vi "Calabro_10566859.vi"() -> ()   [LabVIEW 2017]
uses:
  <vilib>/sound2/lvsound2.llb/Sound Data Format.ctl
  <vilib>/sound2/lvsound2.llb/Sampling Mode.ctl
  <extravilib>/ChannelInstances/Stream-a[.](wfm(dbl))/Read With Abort.vi
  <extravilib>/ChannelInstances/Stream-a[.](wfm(dbl))/Write With Abort.vi
  <extravilib>/ChannelInstances/Stream-a[.](wfm(dbl))/EndpointRead.vi
  <extravilib>/ChannelInstances/Stream-a[.](wfm(dbl))/Endpoint.vi
  <vilib>/sound2/lvsound2.llb/Sound Output Write (DBL Single).vi
  <vilib>/sound2/lvsound2.llb/Sound File Write Open.vi
  <extravilib>/ChannelInstances/Stream-a[.](wfm(dbl))/Instantiate.vi
  <extravilib>/ChannelInstances/Stream-a[.](wfm(dbl))/)Channel.vi
  <resource>/ChannelSupport/_ChannelSupport/WaitIfNeeded.vi
  <vilib>/sound2/lvsound2.llb/Sound File Write (DBL).vi
  <vilib>/measure/matone.llb/Extract Single Tone Information N Chan.vi
  <vilib>/sound2/lvsound2.llb/Sound Input Read (DBL).vi
  <vilib>/measure/NI_MABase.lvlib
  <extravilib>/ChannelInstances/Stream-a[.](wfm(dbl)).lvlib
  <vilib>/measure/NI_MAPro.lvlib
panel:
  in  ".WAV file path":path
  in  "Save audio":bool
  out "Acquired sig. frequency":dbl[](array[numeric]) format="%.2p"
  out "Generated sinusoid":waveform(dbl)(graph)
  in  "Sinusoid generation":bool
  in  "Amplitude (V)":dbl(slide) scale=0.0..10.0
  in  "Frequency (Hz)":dbl(knob) scale=0.0..10000.0
  out "Acquired Audio Graph":waveform(dbl)[](graph)
  in  "stop":bool
  # "Name: Davide Calabrò\nPerson Code: 10566859\nMatricola: 944490"
  # "Exercise 1"
  # "I assume the amplitude expressed in\nvolts (V). I don't know how my sound\ncard manages it."
  # "Exercise 2"
  # "In this exercise I also add a waveform graph\njust to visualize the created sinusoid"
  # "Exercise 3"
  # "Exercise 4"
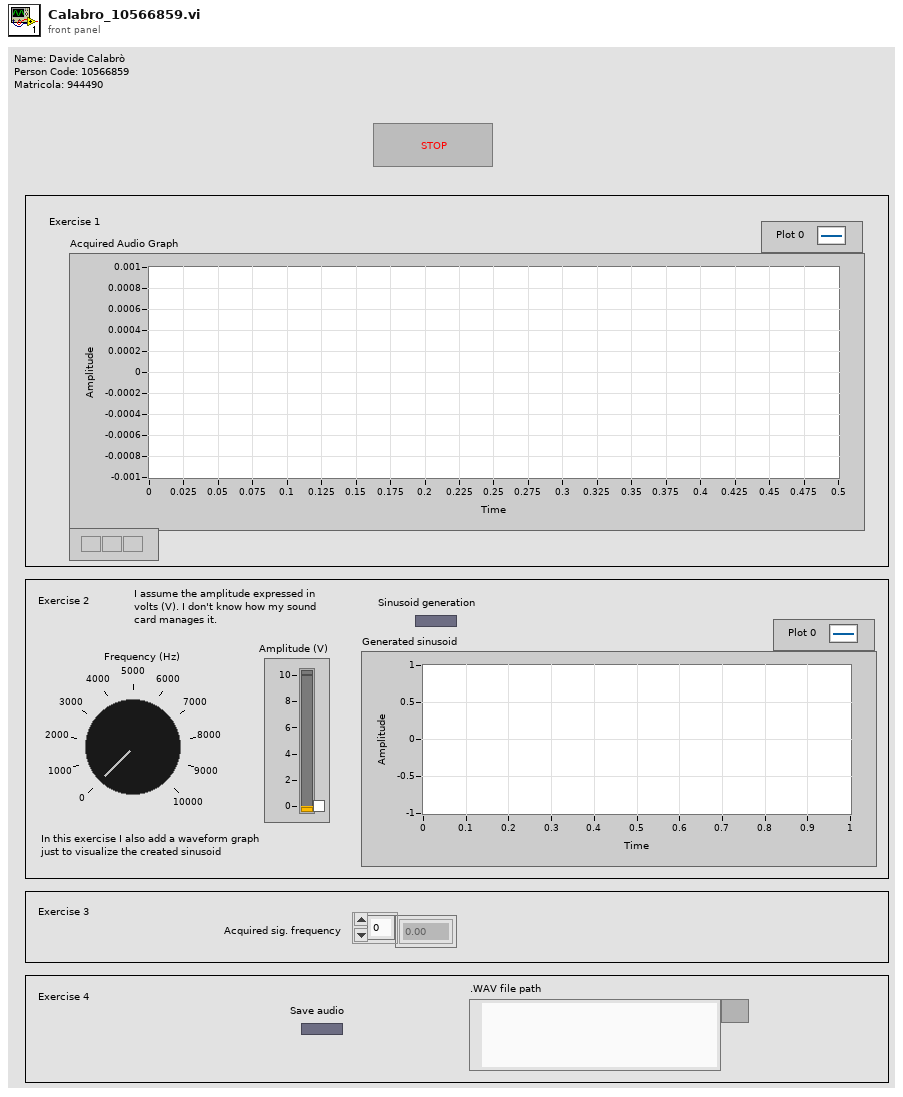
[diagram p1: front panel]
types:
  T1 = typedef "Sound Data Format.ctl" = cluster{"sample rate (S/s)":dbl, "number of channels":i32, "bits per sample":i32}
  T2 = typedef "Sampling Mode.ctl" = i32
  T3 = typedef "Sound File Refnum.ctl" = refnum<file>
  T4 = typedef "Sound Input Task ID.ctl" = u32
  T5 = typedef "Sound Output Task ID.ctl" = u32
  T6 = typedef "Stream-a[.](wfm(dbl)).lvlib/)Channel.ctl" = refnum<queue>
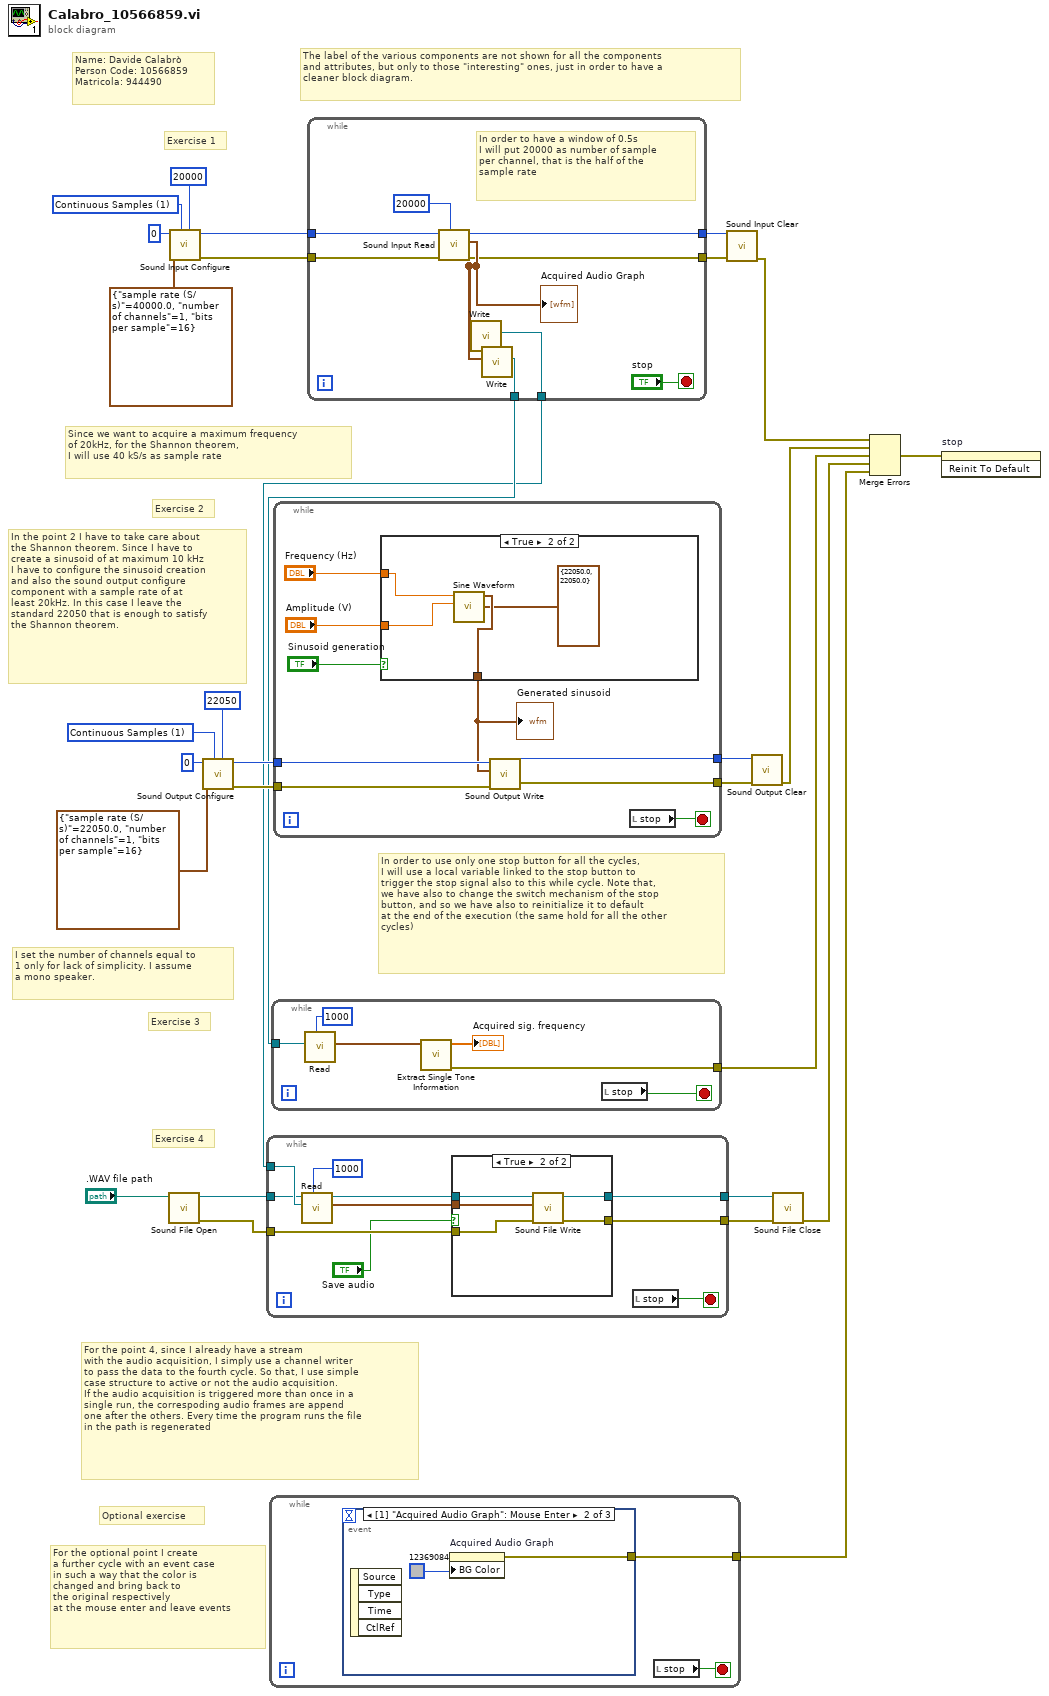
[diagram p0: block diagram]
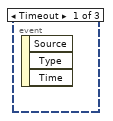
[diagram p2: hidden frame]
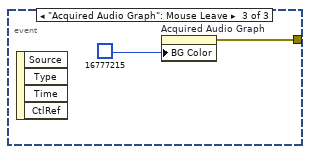
[diagram p3: hidden frame]
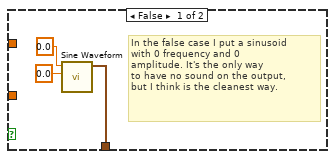
[diagram p5: hidden frame]
diagram:
  w18 = T2 1 items=["Finite Samples", "Continuous Samples"] ("sample mode")
  w27 = T2 1 items=["Finite Samples", "Continuous Samples"] ("sample mode")
  # "The label of the various components are not shown for all the components\nand attributes, but only to those \"interesting\" ones, just in order to have a\ncleaner block diagram."
  # "In the point 2 I have to take care about\nthe Shannon theorem. Since I have to \ncreate a sinusoid of at maximum 10 kHz\nI have to configure the sinusoid creation\nand also the sound output configure\ncomponent with a sample rate of at\nleast 20kHz. In this case I leave the\nstandard 22050 that is enough to satisfy\nthe Shannon theorem."
  # "For the optional point I create\na further cycle with an event case\nin such a way that the color is \nchanged and bring back to \nthe original respectively\nat the mouse enter and leave events"
  # "Optional exercise"
  # "For the point 4, since I already have a stream \nwith the audio acquisition, I simply use a channel writer\nto pass the data to the fourth cycle. So that, I use simple\ncase structure to active or not the audio acquisition.\nIf the audio acquisition is triggered more than once in a\nsingle run, the correspoding audio frames are append\none after the others. Every time the program runs the file\nin the path is regenerated"
  # "Exercise 4"
  # "Exercise 3"
  # "I set the number of channels equal to\n1 only for lack of simplicity. I assume\na mono speaker."
  # "In order to use only one stop button for all the cycles,\nI will use a local variable linked to the stop button to\ntrigger the stop signal also to this while cycle. Note that,\nwe have also to change the switch mechanism of the stop\nbutton, and so we have also to reinitialize it to default\nat the end of the execution (the same hold for all the other\ncycles)"
  # "Exercise 2"
  # "Since we want to acquire a maximum frequency\nof 20kHz, for the Shannon theorem, \nI will use 40 kS/s as sample rate"
  # "Exercise 1"
  # "Name: Davide Calabrò\nPerson Code: 10566859\nMatricola: 944490"
  n1 = call-poly <vilib>:"Sound File Open.vi"("path"=".WAV file path") -> ("error out"=w2:errorcluster, "sound file refnum"=w6:T3)  [unwired: 9 in]
  n2 = call <vilib>:"Sound Input Configure.vi"("number of samples/ch"=20000, "sample mode"=w27, "sound format"=T1 {"sample rate (S/s)"=40000.0, "number of channels"=1, "bits per sample"=16}, "device ID"=u32 0) -> ("error out"=w24:errorcluster, "task ID"=w25:T4)  [unwired: 6 in]
  n3 = call <vilib>:"Sound Output Configure.vi"("number of samples/ch"=22050, "sample mode"=w18, "sound format"=T1 {"sample rate (S/s)"=22050.0, "number of channels"=1, "bits per sample"=16}, "device ID"=u32 0) -> ("error out"=w14:errorcluster, "task ID"=w15:T5)  [unwired: 6 in]
  n4 = while {
    tunnel: [w30] -> w1
    stop <- w31 stop-if-true
    n5 = event shown="[1] \"Acquired Audio Graph\": Mouse Enter" {
      selector: _ -> [_ _ _]
      dyn-events: _ -> [_ _ _]
      timeout: _ -> [_ _ _]
      tunnel: [_ w33 w35] -> w30
      event Timeout {
        n6 = event-data() -> ()  [unwired: 1 in, 3 out]
      }
      event "Acquired Audio Graph": Mouse Enter {
        n7 = event-data() -> ()  [unwired: 1 in, 4 out]
        n8 = property on="Acquired Audio Graph" class="WFGraph (strict)"("BG Color"=u32 12369084) -> (error out=w33:errorcluster)  [unwired: 2 in, 1 out]
      }
      event "Acquired Audio Graph": Mouse Leave {
        n9 = event-data() -> ()  [unwired: 1 in, 4 out]
        n10 = property on="Acquired Audio Graph" class="WFGraph (strict)"("BG Color"=u32 16777215) -> (error out=w35:errorcluster)  [unwired: 2 in, 1 out]
      }
    }
    n11 = local read "stop"() -> (w31:bool)
  }
  n12 = while {
    tunnel: w15 -> [w40]
    tunnel: w14 -> [w39]
    tunnel: [w38] -> w13
    tunnel: [w37] -> w12
    stop <- w44 stop-if-true
    n13 = case shown="True" "Sinusoid generation" {
      tunnel: "Frequency (Hz)" -> [_ w51]
      tunnel: "Amplitude (V)" -> [_ w50]
      tunnel: [w47 w49] -> w36
      frame False {
        # "In the false case I put a sinusoid\nwith 0 frequency and 0 \namplitude. It's the only way\nto have no sound on the output,\nbut I think is the cleanest way."
        n14 = call <vilib>:"Sine Waveform.vi"("amplitude"=0.0, "frequency"=0.0) -> ("signal out"=w47:waveform(dbl))  [unwired: 8 in, 1 out]
      }
      frame True {
        n15 = call <vilib>:"Sine Waveform.vi"("sampling info"=cluster{"Fs":dbl, "#s":dbl} {"Fs"=22050.0, "#s"=22050.0}, "amplitude"=w50, "frequency"=w51) -> ("signal out"=w49:waveform(dbl))  [unwired: 7 in, 1 out]
      }
    }
    "Generated sinusoid" <- w36
    n16 = call-poly <vilib>:"Sound Output Write.vi"("error in (no error)"=w39, "data"=w36, "task ID"=w40) -> ("error out"=w37:errorcluster, "task ID out"=w38:T5)  [unwired: 7 in]
    n17 = local read "stop"() -> (w44:bool)
  }
  n18 = while {
    tunnel: w25 -> [w59]
    tunnel: w24 -> [w58]
    tunnel: [w55] -> w23
    tunnel: [w54] -> w22
    tunnel: [w53] -> w10
    tunnel: [w52] -> w8
    stop <- "stop" stop-if-true
    # "In order to have a window of 0.5s\nI will put 20000 as number of sample\nper channel, that is the half of the\nsample rate"
    n19 = call-poly <vilib>:"Sound Input Read.vi"("number of samples/ch"=20000, "error in (no error)"=w58, "task ID"=w59) -> ("error out"=w54:errorcluster, "data"=w56:waveform(dbl)[], "task ID out"=w55:T4)  [unwired: 6 in]
    "Acquired Audio Graph" <- w56
    n20 = call <extravilib>:"Write.vi"("element"=w56) -> ("channel"=w52:T6)  [unwired: 8 in, 2 out]
    n21 = call <extravilib>:"Write.vi"("element"=w56) -> ("channel"=w53:T6)  [unwired: 8 in, 2 out]
  }
  n22 = while {
    tunnel: w8 -> [w69]
    tunnel: w6 -> [w67]
    tunnel: [w66] -> w5
    tunnel: [w64] -> w3
    tunnel: w2 -> [w63]
    stop <- w65 stop-if-true
    n23 = call <extravilib>:"Read.vi"("timeout in ms (-1)"=1000, "channel"=w69) -> ("element"=w68:waveform(dbl)[])  [unwired: 5 in, 4 out]
    n24 = case shown="True" "Save audio" {
      tunnel: w68 -> [_ w76]
      tunnel: w67 -> [w71 w75]
      tunnel: [w71 w74] -> w66
      tunnel: [w70 w73] -> w64
      tunnel: w63 -> [w70 w72]
      frame False {
      }
      frame True {
        n25 = call-poly <vilib>:"Sound File Write.vi"("error in (no error)"=w72, "data"=w76, "sound file refnum"=w75) -> ("error out"=w73:errorcluster, "sound file refnum out"=w74:T3)  [unwired: 7 in]
      }
    }
    n26 = local read "stop"() -> (w65:bool)
  }
  n27 = while {
    tunnel: w10 -> [w82]
    tunnel: [w77] -> w9
    stop <- w78 stop-if-true
    n28 = call <extravilib>:"Read.vi"("timeout in ms (-1)"=1000, "channel"=w82) -> ("element"=w81:waveform(dbl)[])  [unwired: 5 in, 4 out]
    n29 = call-poly <vilib>:"Extract Single Tone Information.vi"("time signals in"=w81) -> ("error out"=w77:errorcluster, "detected frequencies"=→"Acquired sig. frequency":dbl[])  [unwired: 5 in, 4 out]
    n30 = local read "stop"() -> (w78:bool)
  }
  n31 = call <vilib>:"Sound Input Clear.vi"("error in (no error)"=w22, "task ID"=w23) -> ("error out"=w21:errorcluster)  [unwired: 9 in]
  n32 = call <vilib>:"Sound Output Clear.vi"("error in (no error)"=w12, "task ID"=w13) -> ("error out"=w11:errorcluster)  [unwired: 9 in]
  n33 = call <vilib>:"Sound File Close.vi"("error in (no error)"=w3, "sound file refnum"=w5) -> ("error out"=w4:errorcluster)  [unwired: 9 in]
  n34 = Merge Errors(w21, w11, w9, w4, w1) -> (w20:errorcluster)
  n35 = invoke on="stop" class="Bool (strict)" method="Reinit To Default"(error in=w20) -> ()  [unwired: 2 in, 3 out]
